vi "H5Pget_hyper_vector_size.vi"(6 "error in (no error)":errorcluster, 9 "HDF5 Property Ref":T1) -> (0 "error out":errorcluster, 2 "Vector Size":u32=1024 min=2 step=1, 3 "HDF5 Ref out":T1)   [LabVIEW 2017]
doc: "Retrieves number of I/O vectors to be read/written in hyperslab I/O."
uses:
  <vilib>/UPVI/lvhdf5/library.llb/HDF5 Ref.ctl
  <vilib>/UPVI/lvhdf5/hdf5.dll
panel:
  # "LVHDF5 Toolkit\nCopyright (c) 2005-2013 by Jason D. Sommerville\nCopyright (c) 2014 by UPVI, LLC.\n\nThis use and distribution of this file is governed by the terms found in \nLICENSE.txt distributed with this toolkit and installed at\n <user.lib>\\_lvhdf5\\LICENSE.txt"
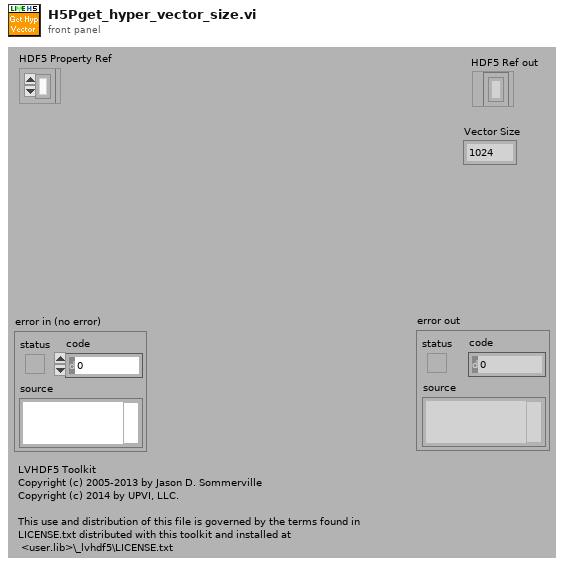
[diagram p1: front panel]
types:
  T1 = typedef "HDF5 Ref.ctl" = refnum<k1>
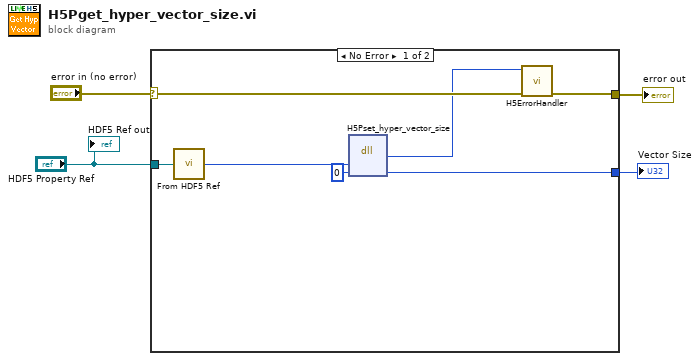
[diagram p0: block diagram]
diagram:
  n1 = case shown="No Error" "error in (no error)" {
    selector: "error in (no error)" -> [w11 w12]
    tunnel: [w10 w12] -> w3
    tunnel: "HDF5 Property Ref" -> [w8 _]
    tunnel: [w6 _] -> w1
    frame No Error {
      n2 = call <vilib>:"From HDF5 Ref.vi"("HDF5 Ref"=w8) -> ("I32"=w7:i32)
      n3 = dll-call lib="C:/Program Files/National Instruments/LabVIEW 2017/vi.lib/UPVI/lvhdf5/hdf5.dll" fn="H5Pset_hyper_vector_size" label="H5Pget_hyper_vector_size"("plist_id"=w7, "vector_size"=u32 0) -> ("return type"=w9:u32, "vector_size"=w6:u64)  [unwired: 4 in, 2 out]
      n4 = call <vilib>:"H5ErrorHandler.vi"("error in (no error)"=w11, "herr_t"=w9) -> ("error out"=w10:errorcluster)  [unwired: 3 in, 4 out]
    }
    frame Error {
    }
  }
  "error out" <- w3
  "Vector Size" <- w1
  "HDF5 Ref out" <- "HDF5 Property Ref"
